vi "SC tester interface v1.vi"() -> ()   [LabVIEW 2011]
doc: "This VI demonstrates how to set up a GPIB board as a non system controller to simulate an instrument using the following steps:\n\nOpen a VISA session to the GPIB interface, set it as the non-system controller, and assign it a primary address. \nUse the VISA Enable Event VI to register the \"GPIB Listener\" Event; this event occurs when the GPIB interface is addressed as a listener. \nUse the VISA Wait on Event VI to wait until the GPIB interface is a listener; this means that there is data available on the bus for the interface.\nUse the VISA Read VI to read the available data, parse it, and send an appropriate response.\nCall the VISA close VI after the stop button is pressed\n\nNote: For a description of other available VISA event types, see the NI-VISA help."
uses:
  GPIB/handler GPIBsim/SC virtual handler states.ctl
  <vilib>/Instr/_visa.llb/Select Event Type.ctl
panel:
  out "tester measured index time":u32
  out "tester it end hidden":u32
  out "tester it start hidden":u32
  out "tester measured wait time":u32
  out "tester wt end hidden":u32
  out "tester wt start hidden":u32
  out "tester measured test time":u32
  out "tester tt end hidden":u32
  out "tester tt start hidden":u32
  in  "devices ready hidden":string
  in  "binning_string hidden":string
  out "VISA bus 0 resource name out":refnum<visa-resource-name>
  out "VISA bus 0 error out":errorcluster
  in  "SC virtual handler states":T1
  out "VISA close error":bool
  out "VISA open error":bool
  out "gpib read error":bool
  out "gpib write error":bool
  out "on-line test time":dbl=0.1 min=0.1 max=50.0 step=0.1 format="%.2f"
  out "tester indexing":bool
  out "tester testing":bool
  out "Good devices":u64
  out "devices tested":u64
  out "yiereld":dbl format="%#.0f"
  in  "handler listens to tester at":refnum<visa-resource-name>="GPIB1::INTFC"
  out "message received from Sentinel Controller":string
  out "Message sent to Sentinel Controller":string
  in  "parallelism reported by handler":u8
  out "parallelism mismatch":bool
  # "Celerint Sentinel Controller ~ Handler Simulator"
  # "`"
  # "GPIB address is 1 on this laptop"
  # "%"
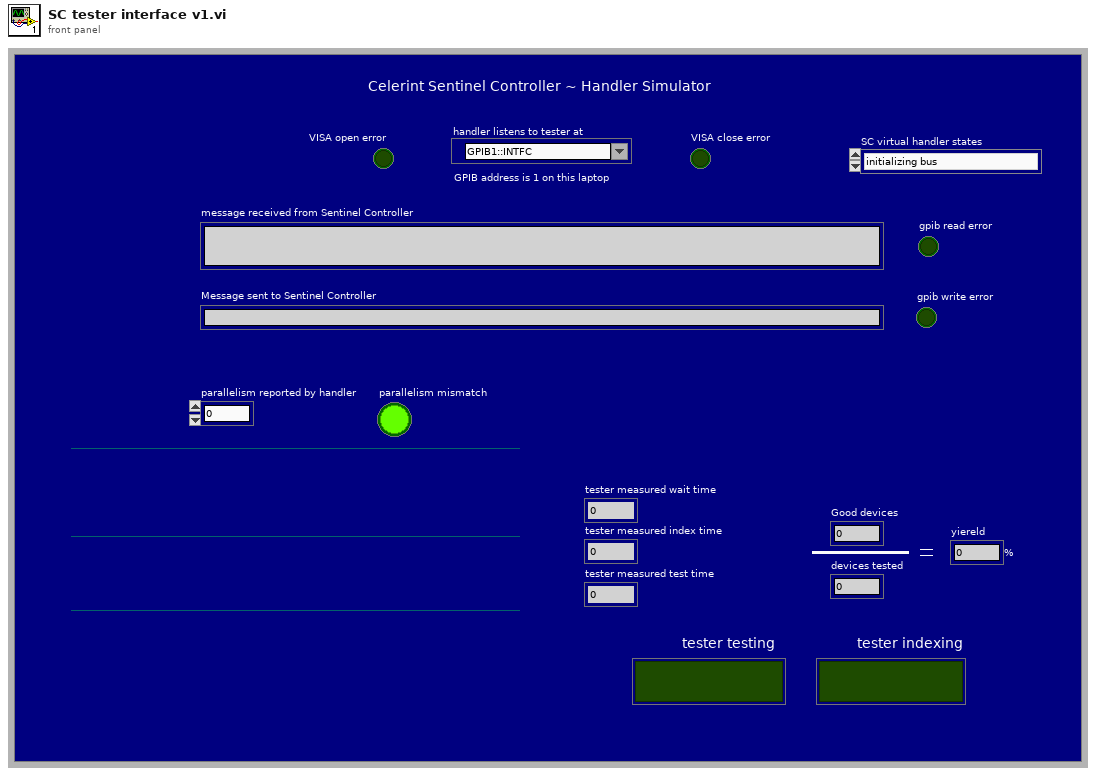
[diagram p1: front panel]
types:
  T1 = typedef "SC virtual handler states.ctl" = enum16{"initializing bus", "waiting on event", "reading", "responding to *SITES?", "responding to *IDN?", "respond to *HAND?", "redponding to *HF", "responding to *HS", "testing", "indexing", "responding to unknown command", "closing bus"}
  T2 = typedef "Select Event Type.ctl" = u32
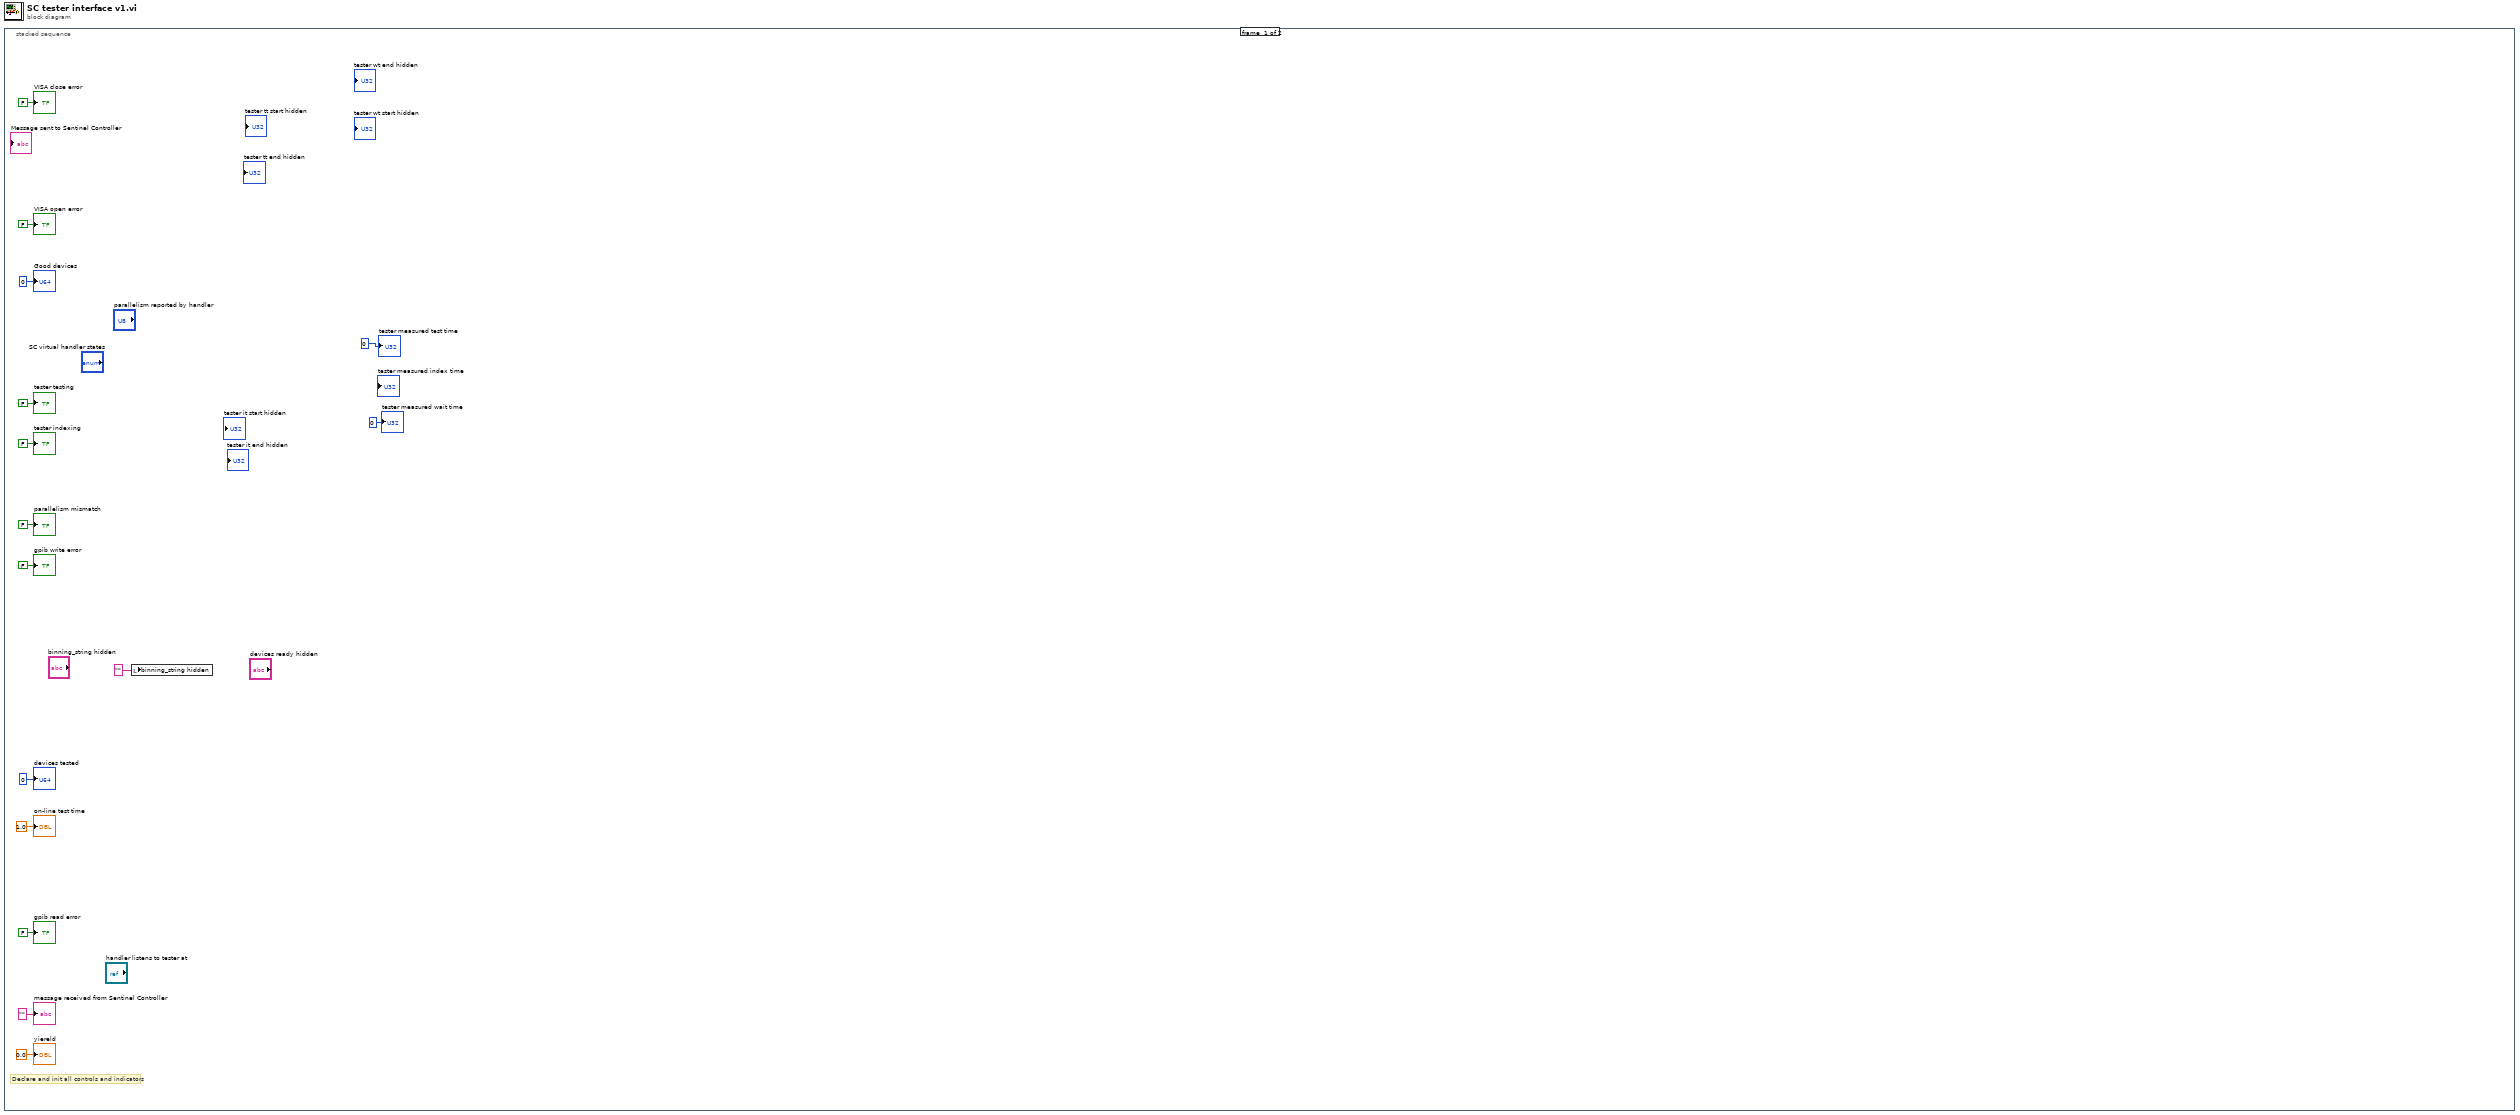
[diagram p0: block diagram]
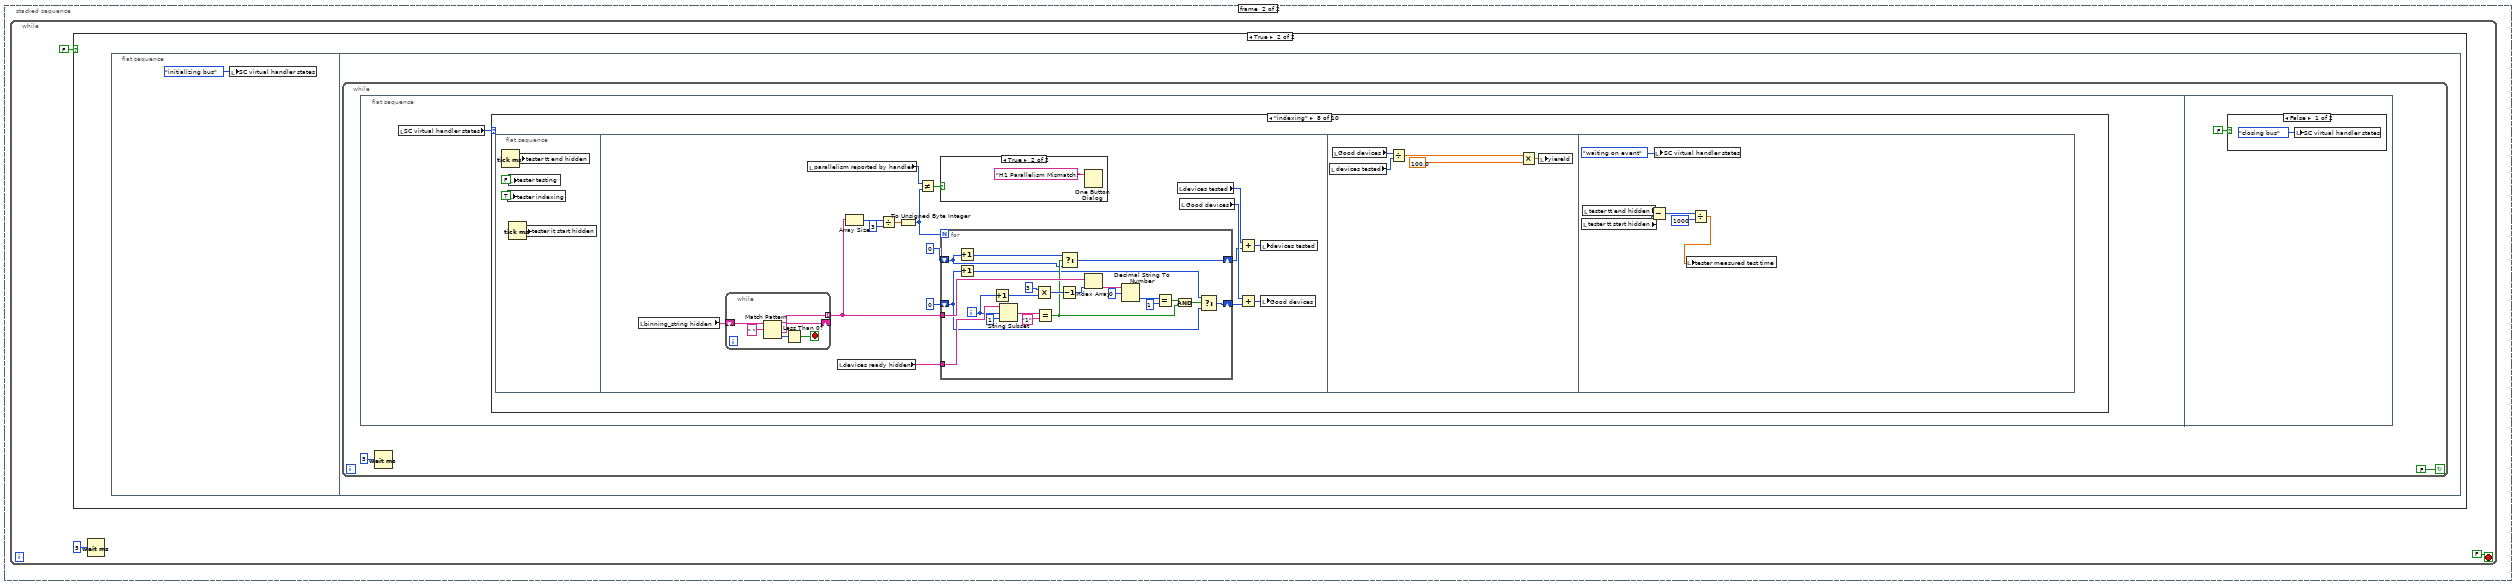
[diagram p2: hidden frame]
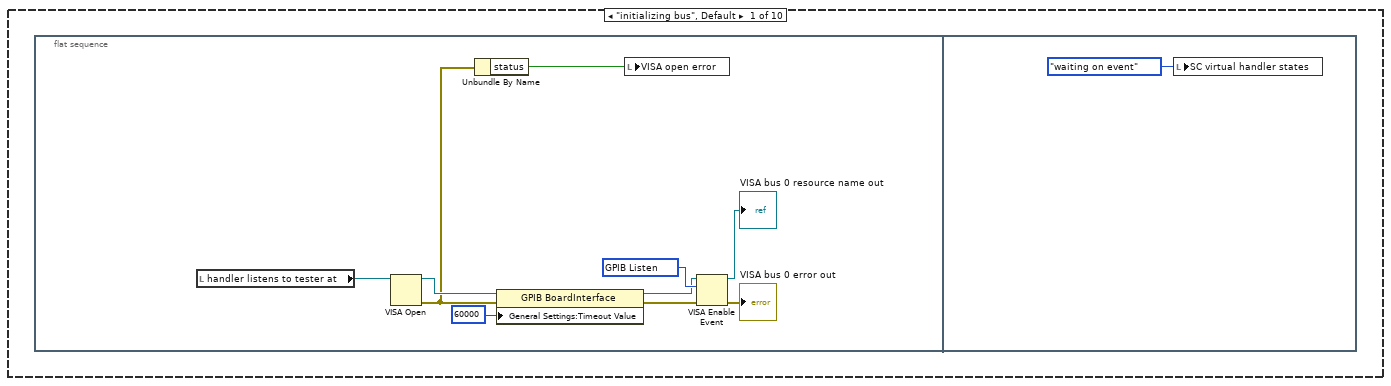
[diagram p4: hidden frame]
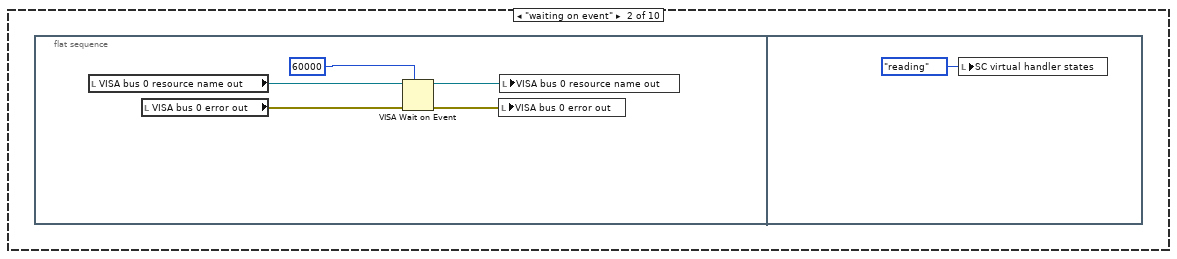
[diagram p5: hidden frame]
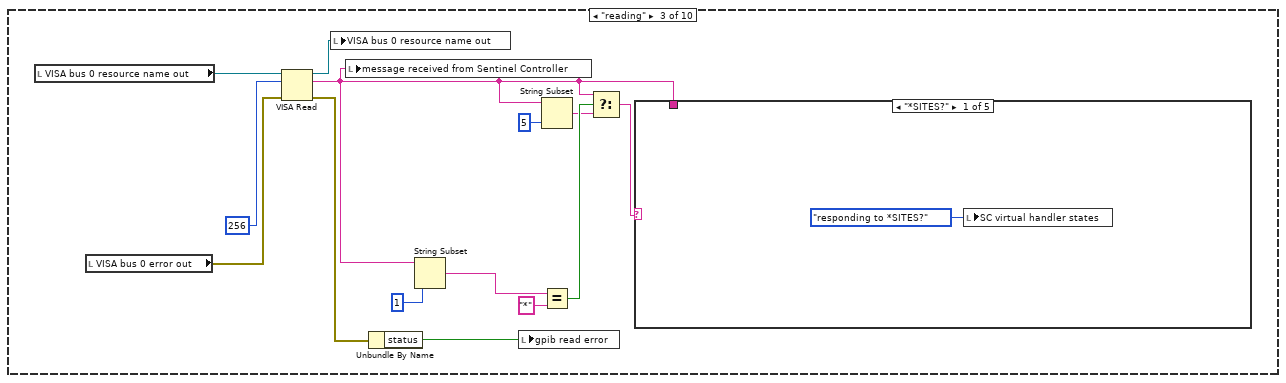
[diagram p6: hidden frame]
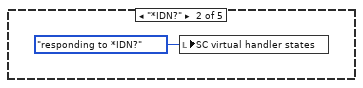
[diagram p7: hidden frame]
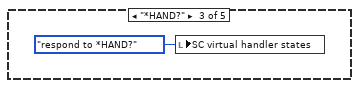
[diagram p8: hidden frame]
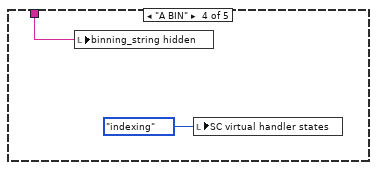
[diagram p9: hidden frame]
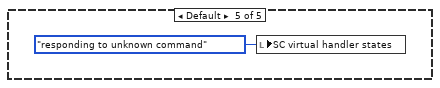
[diagram p10: hidden frame]
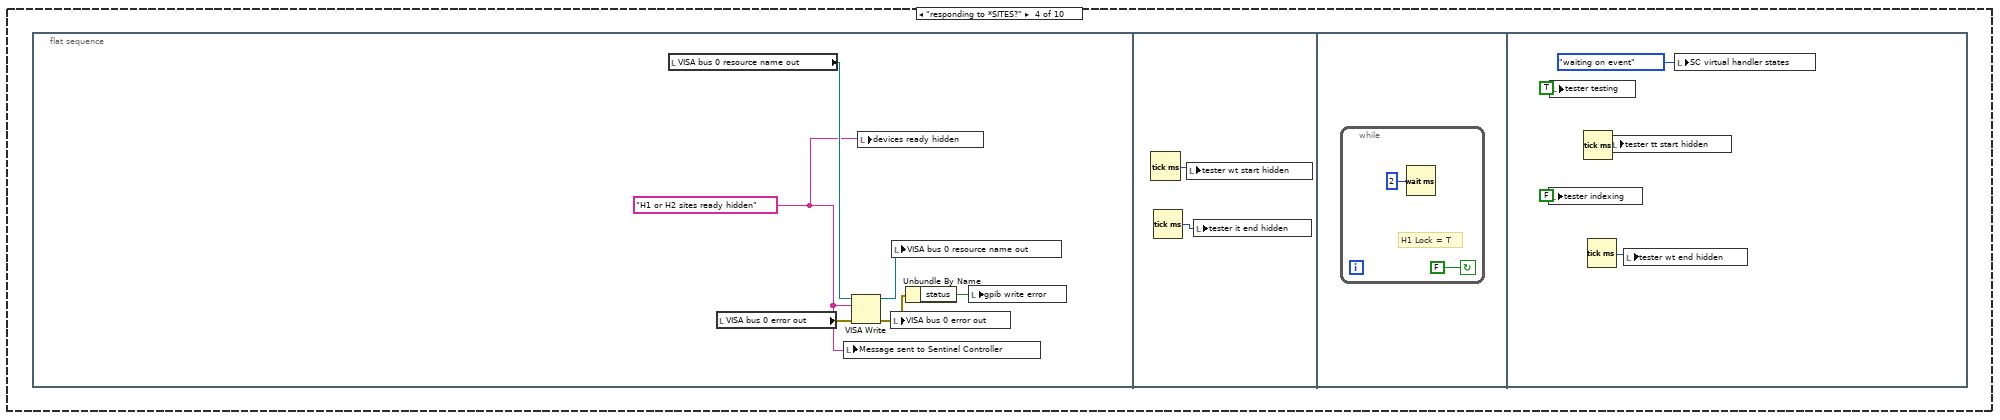
[diagram p11: hidden frame]
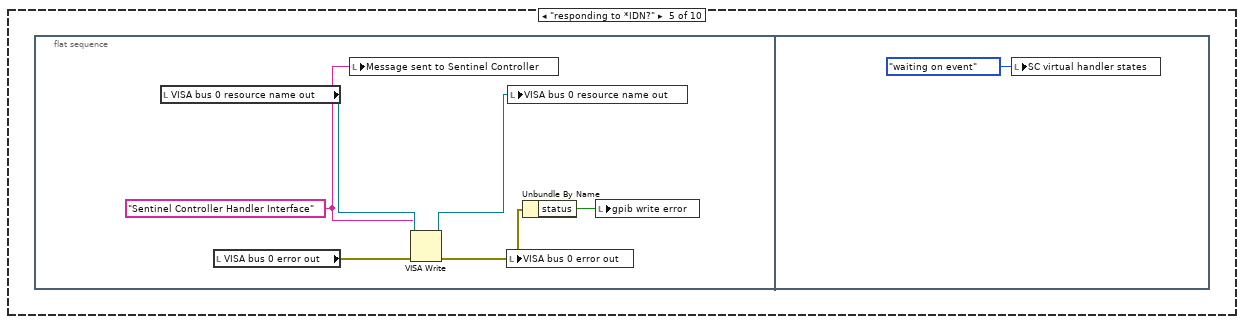
[diagram p12: hidden frame]
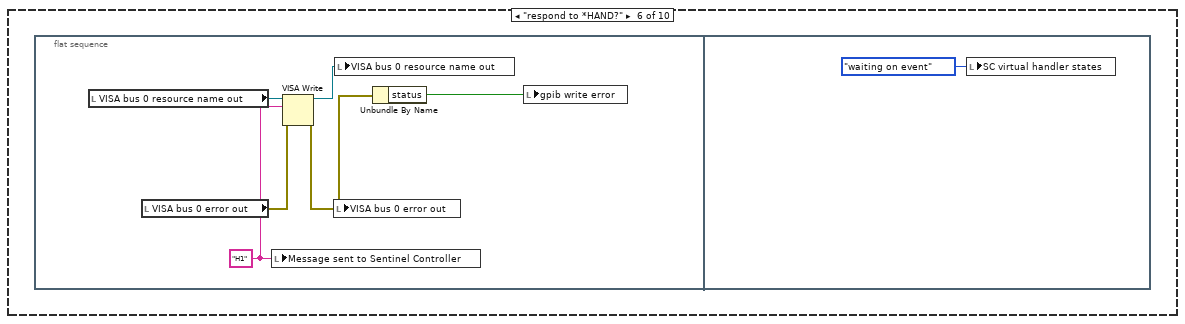
[diagram p13: hidden frame]
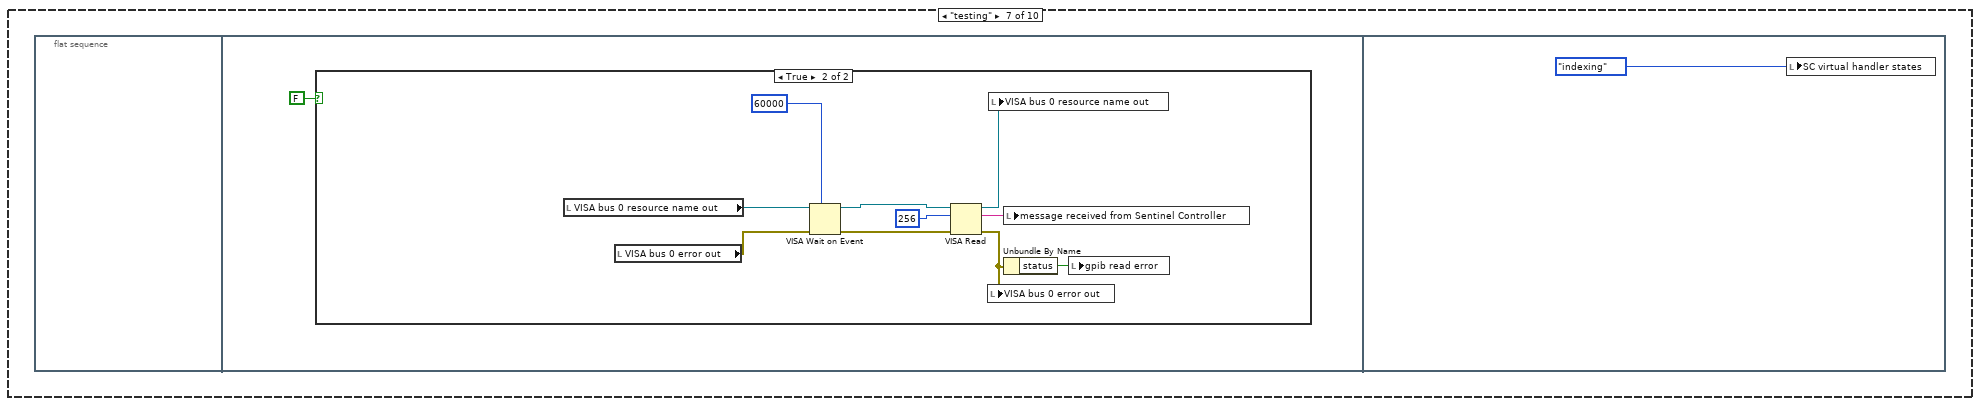
[diagram p14: hidden frame]
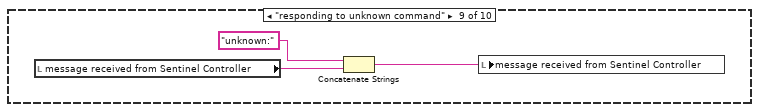
[diagram p17: hidden frame]
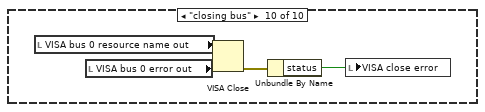
[diagram p18: hidden frame]
diagram:
  n1 = stacked-sequence {
    frame #0 {
      # "Declare and init all controls and indicators"
      n2 = local write "binning_string hidden"("" ("binning_string")) -> ()
      "Good devices" <- u64 0 ("Good Devices")
      "devices tested" <- u64 0 ("Devices Tested")
      "yiereld" <- 0.0 ("Yield")
      "tester indexing" <- FALSE ("Indexing")
      "tester testing" <- FALSE ("Testing")
      "message received from Sentinel Controller" <- "" ("Message received from Sentinel Controller")
      "parallelism mismatch" <- FALSE ("Parallelism mismatch")
      "on-line test time" <- 1.0 ("On-line test time")
      "gpib write error" <- FALSE ("GPIB write error")
      "gpib read error" <- FALSE ("GPIB read error")
      "VISA close error" <- FALSE ("VISA close error")
      "VISA open error" <- FALSE ("VISA open error")
      "tester measured test time" <- u32 0 ("Measured test time")
      "tester measured wait time" <- u32 0 ("Measured wait time")
    }
    frame #1 {
      n3 = while {
        stop <- FALSE stop-if-true
        n4 = case shown="True" FALSE {
          frame False {
          }
          frame True {
            n5 = flat-sequence {
              frame #0 {
                n6 = local write "SC virtual handler states"(SC_virtual_handler_states."initializing bus" ("SC Test Interface States")) -> ()
              }
              frame #1 {
                n7 = while {
                  stop <- FALSE continue-if-true
                  n8 = flat-sequence {
                    frame #0 {
                      n9 = local read "SC virtual handler states"() -> (w22:T1)
                      n10 = case shown="\"indexing\"" w22 {
                        frame "initializing bus", Default {
                          n11 = flat-sequence {
                            frame #0 {
                              w29 = T2 1073684500 items=["Service Request"=1073684491, "Trigger"=3221168138, "Clear"=1073684493, "VXI Signal"=1073684512, "VXI/VME Interrupt"=3221168161, "VXI/VME Sysfail"=1073684509, "VXI/VME Sysreset"=1073684510, "GPIB CIC"=1073684498, "GPIB Talk"=1073684499, "GPIB Listen"=1073684500, "PXI Interrupt"=1073684514, "Serial Break"=1073684515, "Serial TermChar"=1073684516, "Serial CTS"=1073684521, "Serial DSR"=1073684522, "Serial DCD"=1073684524, "Serial RI"=1073684526, "Serial Character"=1073684533, "USB Interrupt"=1073684535, "All Enabled"=1073709055] ("Event Type")
                              n12 = local read "handler listens to tester at"() -> (w25:refnum<visa-resource-name>)
                              n13 = VISA Open(VISA resource name=w25) -> (VISA resource name=w31:refnum<visa-resource-name>, error out=w30:errorcluster)  [unwired: 1 in, 3 out]
                              n14 = Unbundle By Name(w30) -> ("status"=w32:bool)
                              n15 = property class="GPIB BoardInterface"(reference=w31, error in=w30, "General Settings:Timeout Value"=u32 60000) -> (reference out=w28:refnum<visa-resource-name>, error out=w27:errorcluster)
                              n16 = local write "VISA open error"(w32) -> ()
                              n17 = VISA Enable Event(8:w27, 10:w29, 11:w28) -> (0:→"VISA bus 0 error out":errorcluster, 3:→"VISA bus 0 resource name out":refnum<visa-resource-name>)  [unwired: 1 out]
                            }
                            frame #1 {
                              n18 = local write "SC virtual handler states"(SC_virtual_handler_states."waiting on event" ("SC Test Interface States")) -> ()
                            }
                          }
                        }
                        frame "waiting on event" {
                          n19 = flat-sequence {
                            frame #0 {
                              n20 = local read "VISA bus 0 resource name out"() -> (w37:refnum<visa-resource-name>)
                              n21 = local read "VISA bus 0 error out"() -> (w36:errorcluster)
                              n22 = VISA Wait on Event(7:60000, 8:w36, 11:w37) -> (0:w34:errorcluster, 3:w35:refnum<visa-resource-name>)  [unwired: 2 in, 2 out]
                              n23 = local write "VISA bus 0 error out"(w34) -> ()
                              n24 = local write "VISA bus 0 resource name out"(w35) -> ()
                            }
                            frame #1 {
                              n25 = local write "SC virtual handler states"(SC_virtual_handler_states."reading" ("SC Test Interface States")) -> ()
                            }
                          }
                        }
                        frame "reading" {
                          n26 = local read "VISA bus 0 resource name out"() -> (w42:refnum<visa-resource-name>)
                          n27 = local read "VISA bus 0 error out"() -> (w43:errorcluster)
                          n28 = VISA Read(VISA resource name=w42, byte count=256, error in (no error)=w43) -> (VISA resource name out=w41:refnum<visa-resource-name>, read buffer=w40:string, error out=w44:errorcluster)  [unwired: 1 out]
                          n29 = local write "VISA bus 0 resource name out"(w41) -> ()
                          n30 = local write "message received from Sentinel Controller"(w40) -> ()
                          n31 = Unbundle By Name(w44) -> ("status"=w53:bool)
                          n32 = String Subset(string=w40, length (rest)=1 ("length (rest)")) -> (substring=w50:string)  [unwired: 1 in]
                          n33 = local write "gpib read error"(w53) -> ()
                          n34 = String Subset(string=w40, length (rest)=5 ("length (rest)")) -> (substring=w46:string)  [unwired: 1 in]
                          n35 = Equal?(x=w50, y="*") -> (x = y?=w49:bool)
                          n36 = Select(t=w40, s=w49, f=w46) -> (s? t:f=w45:string)
                          n37 = case shown="\"*SITES?\"" w45 {
                            tunnel: w40 -> [_ _ _ w57 _]
                            frame "*SITES?" {
                              n38 = local write "SC virtual handler states"(SC_virtual_handler_states."responding to *SITES?" ("SC Test Interface States")) -> ()
                            }
                            frame "*IDN?" {
                              n39 = local write "SC virtual handler states"(SC_virtual_handler_states."responding to *IDN?" ("SC Test Interface States")) -> ()
                            }
                            frame "*HAND?" {
                              n40 = local write "SC virtual handler states"(SC_virtual_handler_states."respond to *HAND?" ("SC Test Interface States")) -> ()
                            }
                            frame "A BIN" {
                              n41 = local write "binning_string hidden"(w57) -> ()
                              n42 = local write "SC virtual handler states"(SC_virtual_handler_states."indexing" ("SC Test Interface States")) -> ()
                            }
                            frame Default {
                              n43 = local write "SC virtual handler states"(SC_virtual_handler_states."responding to unknown command" ("SC Test Interface States")) -> ()
                            }
                          }
                        }
                        frame "responding to *SITES?" {
                          n44 = flat-sequence {
                            frame #0 {
                              w60 = "H1 or H2 sites ready hidden"
                              n45 = local read "VISA bus 0 resource name out"() -> (w63:refnum<visa-resource-name>)
                              n46 = local read "VISA bus 0 error out"() -> (w64:errorcluster)
                              n47 = local write "Message sent to Sentinel Controller"(w60) -> ()
                              n48 = VISA Write(VISA resource name=w63, write buffer=w60, error in (no error)=w64) -> (VISA resource name out=w62:refnum<visa-resource-name>, error out=w61:errorcluster)  [unwired: 1 out]
                              n49 = local write "devices ready hidden"(w60) -> ()
                              n50 = local write "VISA bus 0 error out"(w61) -> ()
                              n51 = local write "VISA bus 0 resource name out"(w62) -> ()
                              n52 = Unbundle By Name(w61) -> ("status"=w65:bool)
                              n53 = local write "gpib write error"(w65) -> ()
                            }
                            frame #1 {
                              n54 = Tick Count (ms)() -> (millisecond timer value=w67:u32)
                              n55 = Tick Count (ms)() -> (millisecond timer value=w66:u32)
                              n56 = local write "tester wt start hidden"(w67) -> ()
                              n57 = local write "tester it end hidden"(w66) -> ()
                            }
                            frame #2 {
                              n58 = while {
                                stop <- FALSE continue-if-true
                                # "H1 Lock = T"
                                n59 = Wait (ms)(milliseconds to wait=u32 2) -> ()  [unwired: 1 out]
                              }
                            }
                            frame #3 {
                              n60 = local write "tester indexing"(FALSE ("indexing")) -> ()
                              n61 = local write "tester testing"(TRUE ("testing")) -> ()
                              n62 = Tick Count (ms)() -> (millisecond timer value=w71:u32)
                              n63 = Tick Count (ms)() -> (millisecond timer value=w70:u32)
                              n64 = local write "tester tt start hidden"(w71) -> ()
                              n65 = local write "tester wt end hidden"(w70) -> ()
                              n66 = local write "SC virtual handler states"(SC_virtual_handler_states."waiting on event" ("SC Test Interface States")) -> ()
                            }
                          }
                        }
                        frame "responding to *IDN?" {
                          n67 = flat-sequence {
                            frame #0 {
                              w75 = "Sentinel Controller Handler Interface"
                              n68 = local read "VISA bus 0 resource name out"() -> (w80:refnum<visa-resource-name>)
                              n69 = local read "VISA bus 0 error out"() -> (w79:errorcluster)
                              n70 = local write "Message sent to Sentinel Controller"(w75) -> ()
                              n71 = VISA Write(VISA resource name=w80, write buffer=w75, error in (no error)=w79) -> (VISA resource name out=w78:refnum<visa-resource-name>, error out=w77:errorcluster)  [unwired: 1 out]
                              n72 = local write "VISA bus 0 error out"(w77) -> ()
                              n73 = local write "VISA bus 0 resource name out"(w78) -> ()
                              n74 = Unbundle By Name(w77) -> ("status"=w76:bool)
                              n75 = local write "gpib write error"(w76) -> ()
                            }
                            frame #1 {
                              n76 = local write "SC virtual handler states"(SC_virtual_handler_states."waiting on event" ("SC Test Interface States")) -> ()
                            }
                          }
                        }
                        frame "respond to *HAND?" {
                          n77 = flat-sequence {
                            frame #0 {
                              w82 = "H1" ("Reply to *IDN? Command")
                              n78 = local read "VISA bus 0 resource name out"() -> (w84:refnum<visa-resource-name>)
                              n79 = local read "VISA bus 0 error out"() -> (w83:errorcluster)
                              n80 = local write "Message sent to Sentinel Controller"(w82) -> ()
                              n81 = VISA Write(VISA resource name=w84, write buffer=w82, error in (no error)=w83) -> (VISA resource name out=w85:refnum<visa-resource-name>, error out=w86:errorcluster)  [unwired: 1 out]
                              n82 = local write "VISA bus 0 error out"(w86) -> ()
                              n83 = local write "VISA bus 0 resource name out"(w85) -> ()
                              n84 = Unbundle By Name(w86) -> ("status"=w87:bool)
                              n85 = local write "gpib write error"(w87) -> ()
                            }
                            frame #1 {
                              n86 = local write "SC virtual handler states"(SC_virtual_handler_states."waiting on event" ("SC Test Interface States")) -> ()
                            }
                          }
                        }
                        frame "testing" {
                          n87 = flat-sequence {
                            frame #0 {
                            }
                            frame #1 {
                              n88 = case shown="True" FALSE {
                                frame False {
                                }
                                frame True {
                                n89 = local read "VISA bus 0 resource name out"() -> (w93:refnum<visa-resource-name>)
                                n90 = local read "VISA bus 0 error out"() -> (w94:errorcluster)
                                n91 = VISA Wait on Event(7:60000, 8:w94, 11:w93) -> (0:w99:errorcluster, 3:w98:refnum<visa-resource-name>)  [unwired: 2 in, 2 out]
                                n92 = VISA Read(VISA resource name=w98, byte count=256, error in (no error)=w99) -> (VISA resource name out=w92:refnum<visa-resource-name>, read buffer=w96:string, error out=w91:errorcluster)  [unwired: 1 out]
                                n93 = local write "VISA bus 0 error out"(w91) -> ()
                                n94 = local write "VISA bus 0 resource name out"(w92) -> ()
                                n95 = local write "message received from Sentinel Controller"(w96) -> ()
                                n96 = Unbundle By Name(w91) -> ("status"=w90:bool)
                                n97 = local write "gpib read error"(w90) -> ()
                                }
                              }
                            }
                            frame #2 {
                              n98 = local write "SC virtual handler states"(SC_virtual_handler_states."indexing" ("SC Test Interface States")) -> ()
                            }
                          }
                        }
                        frame "indexing" {
                          n99 = flat-sequence {
                            frame #0 {
                              n100 = Tick Count (ms)() -> (millisecond timer value=w102:u32)
                              n101 = local write "tester indexing"(TRUE ("indexing")) -> ()
                              n102 = local write "tester testing"(FALSE ("testing")) -> ()
                              n103 = Tick Count (ms)() -> (millisecond timer value=w101:u32)
                              n104 = local write "tester tt end hidden"(w102) -> ()
                              n105 = local write "tester it start hidden"(w101) -> ()
                            }
                            frame #1 {
                              n106 = local read "binning_string hidden"() -> (w117:string)
                              n107 = while {
                                tunnel: [w125] -> w121 mode=indexing
                                shift-right: [w126] -> _
                                shift-left: w117 -> [w128]
                                stop <- w123 stop-if-true
                                n108 = Match Pattern(string=w128, regular expression=" ") -> (before substring=w125:string, after substring=w126:string, offset past match=w124:i32)  [unwired: 2 out]
                                n109 = Less Than 0?(x=w124) -> (x < 0?=w123:bool)
                              }
                              n110 = local read "parallelism reported by handler"() -> (w105:u8)
                              n111 = local read "devices ready hidden"() -> (w112:string)
                              n112 = Array Size(array=w121) -> (size(s)=w118:i32)
                              n113 = Divide(x=w118, y=3) -> (x/y=w120:dbl)
                              n114 = To Unsigned Byte Integer(number=w120) -> (unsigned 8bit integer=w115:u8)
                              n115 = Not Equal?(x=w105, y=w115) -> (x != y?=w116:bool)
                              n116 = case shown="True" w116 {
                                frame False {
                                }
                                frame True {
                                n117 = One Button Dialog(message="H1 Parallelism Mismatch!") -> ()  [unwired: 1 in, 1 out]
                                }
                              }
                              n118 = for {
                                N: w115 -> [_]
                                tunnel: w121 -> [w151]
                                tunnel: w112 -> [w142]
                                shift-right: [w135] -> w108
                                shift-left: 0 -> [w134]
                                shift-right: [w131] -> w106
                                shift-left: 0 -> [w129]
                                i -> [w132]
                                n119 = Increment(x=w134) -> (x+1=w133:i32)
                                n120 = Increment(x=w129) -> (x+1=w130:i32)
                                n121 = Increment(x=w132) -> (x+1=w150:i32)
                                n122 = String Subset(string=w142, offset (0)=w132, length (rest)=1 ("length (rest)")) -> (substring=w138:string)
                                n123 = Multiply(x=3, y=w150) -> (x*y=w144:i32)
                                n124 = Equal?(x=w138, y="1") -> (x = y?=w136:bool)
                                n125 = Decrement(x=w144) -> (x-1=w143:i32)
                                n126 = Select(t=w133, s=w136, f=w134) -> (s? t:f=w135:i32)
                                n127 = Index Array(array=w151, index=w143) -> (element=w148:string)
                                n128 = Decimal String To Number(string=w148, offset=0) -> (number=w146:i32)  [unwired: 1 in, 1 out]
                                n129 = Equal?(x=w146, y=1) -> (x = y?=w139:bool)
                                n130 = And(x=w139, y=w136) -> (x .and. y?=w140:bool)
                                n131 = Select(t=w130, s=w140, f=w129) -> (s? t:f=w131:i32)
                              }
                              n132 = local read "devices tested"() -> (w110:u64)
                              n133 = local read "Good devices"() -> (w113:u64)
                              n134 = Add(x=w110, y=w108) -> (x+y=w109:u64)
                              n135 = Add(x=w113, y=w106) -> (x+y=w114:u64)
                              n136 = local write "devices tested"(w109) -> ()
                              n137 = local write "Good devices"(w114) -> ()
                            }
                            frame #2 {
                              n138 = local read "devices tested"() -> (w155:u64)
                              n139 = local read "Good devices"() -> (w156:u64)
                              n140 = Divide(x=w156, y=w155) -> (x/y=w154:dbl)
                              n141 = Multiply(x=w154, y=100.0) -> (x*y=w153:dbl)
                              n142 = local write "yiereld"(w153) -> ()
                            }
                            frame #3 {
                              n143 = local read "tester tt start hidden"() -> (w160:u32)
                              n144 = local read "tester tt end hidden"() -> (w161:u32)
                              n145 = Subtract(x=w161, y=w160) -> (x-y=w159:u32)
                              n146 = local write "SC virtual handler states"(SC_virtual_handler_states."waiting on event" ("SC Test Interface States")) -> ()
                              n147 = Divide(x=w159, y=u32 1000) -> (x/y=w157:dbl)
                              n148 = local write "tester measured test time"(w157) -> ()
                            }
                          }
                        }
                        frame "responding to unknown command" {
                          n149 = local read "message received from Sentinel Controller"() -> (w164:string)
                          n150 = Concatenate Strings("unknown:", w164) -> (w163:string)
                          n151 = local write "message received from Sentinel Controller"(w163) -> ()
                        }
                        frame "closing bus" {
                          n152 = local read "VISA bus 0 resource name out"() -> (w167:refnum<visa-resource-name>)
                          n153 = local read "VISA bus 0 error out"() -> (w166:errorcluster)
                          n154 = VISA Close(VISA resource name=w167, error in (no error)=w166) -> (error out=w169:errorcluster)
                          n155 = Unbundle By Name(w169) -> ("status"=w168:bool)
                          n156 = local write "VISA close error"(w168) -> ()
                        }
                      }
                    }
                    frame #1 {
                      n157 = case shown="False" FALSE {
                        frame False {
                          n158 = local write "SC virtual handler states"(SC_virtual_handler_states."closing bus" ("SC Test Interface States")) -> ()
                        }
                        frame True {
                        }
                      }
                    }
                  }
                  n159 = Wait (ms)(milliseconds to wait=u32 5) -> ()  [unwired: 1 out]
                }
              }
            }
          }
        }
        n160 = Wait (ms)(milliseconds to wait=u32 5) -> ()  [unwired: 1 out]
      }
    }
  }
